vi "CreateOpenFile.vi"(3 "Prompt String":string="Select a temperature log file.") -> (0 "error out":errorcluster, 1 "refnum out":refnum<file>)   [LabVIEW 2013]
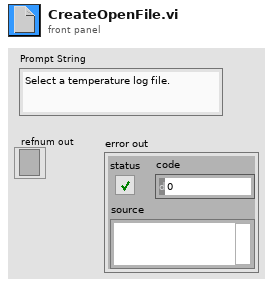
[diagram p1: front panel]
types:
  T1 = enum16{"open", "replace", "create", "open or create", "replace or create", "replace or create with confirmation"}
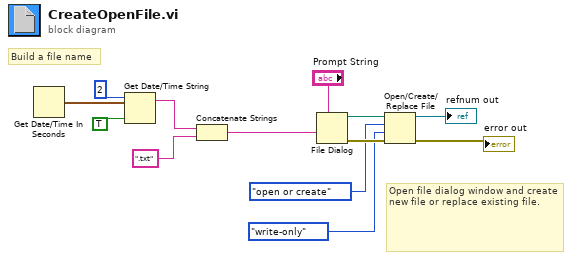
[diagram p0: block diagram]
diagram:
  # "Build a file name"
  # "Open file dialog window and create new file or replace existing file."
  n1 = Get Date/Time In Seconds() -> (seconds since 1Jan1904=w4:timestamp)
  n2 = Get Date/Time String(date format (0)=2, seconds (now)=w4, want seconds? (F)=TRUE) -> (date string=w7:string)  [unwired: 1 out]
  n3 = Concatenate Strings(w7, ".txt") -> (w5:string)
  n4 = File Dialog(7:"Prompt String", 9:w5) -> (0:w12:errorcluster, 3:w13:path)  [unwired: 5 in, 2 out]
  n5 = Open/Create/Replace File(file path (use dialog)=w13, error in=w12, operation (0:open)=T1."open or create", access (0:read/write)=enum16{"read/write", "read-only", "write-only"}."write-only") -> (refnum out=→"refnum out":refnum<file>, error out=→"error out":errorcluster)  [unwired: 2 in, 1 out]
